vi "Wall avoidance robot.vi"() -> ()   [LabVIEW 2018]
uses:
  <vilib>/myRIO/Common/Instrument Driver Framework/myRIO v1.0/AI/typedefs/AI Channels Enum.ctl
  <vilib>/myRIO/Common/Instrument Driver Framework/myRIO v1.0/AI/typedefs/AI Channels List.ctl
panel:
  in  "Boolean":bool
  out "Sharp IR Distance 2":dbl
  out "Sharp IR Distance":dbl
  out "Speed":T1
  out "Distance":T2
  in  "stop":bool
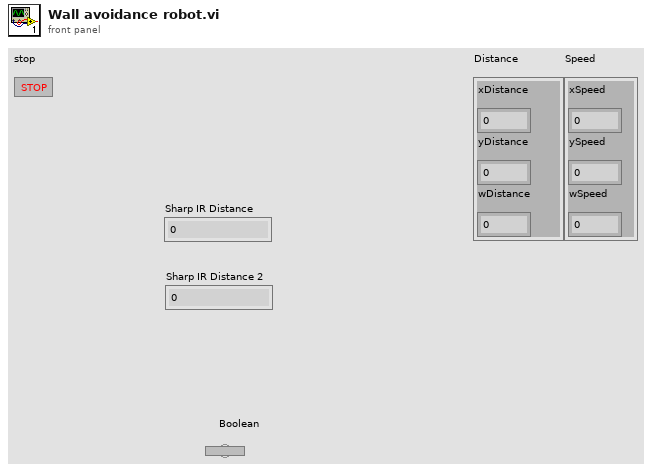
[diagram p1: front panel]
types:
  T1 = cluster{"xSpeed":dbl, "ySpeed":dbl, "wSpeed":dbl}
  T2 = cluster{"xDistance":dbl, "yDistance":dbl, "wDistance":dbl}
  T3 = typedef "AI Channels List.ctl" = T4[]
  T4 = typedef "AI Channels Enum.ctl" = enum16{"Not Connected", "AudioIn/Left", "AudioIn/Right", "C/AI0", "C/AI1", "A/AI0", "A/AI1", "A/AI2", "A/AI3", "A/AI4", "A/AI5", "A/AI6", "A/AI7", "B/AI0", "B/AI1", "B/AI2", "B/AI3", "B/AI4", "B/AI5", "B/AI6", "B/AI7", "AI/AI0", "AI/AI1", "AI/AI2", "AI/AI3", "A/AI0 (DIFF)", "A/AI1 (DIFF)", "A/AI2 (DIFF)", "A/AI3 (DIFF)", "B/AI0 (DIFF)", "B/AI1 (DIFF)", "B/AI2 (DIFF)", "B/AI3 (DIFF)"}
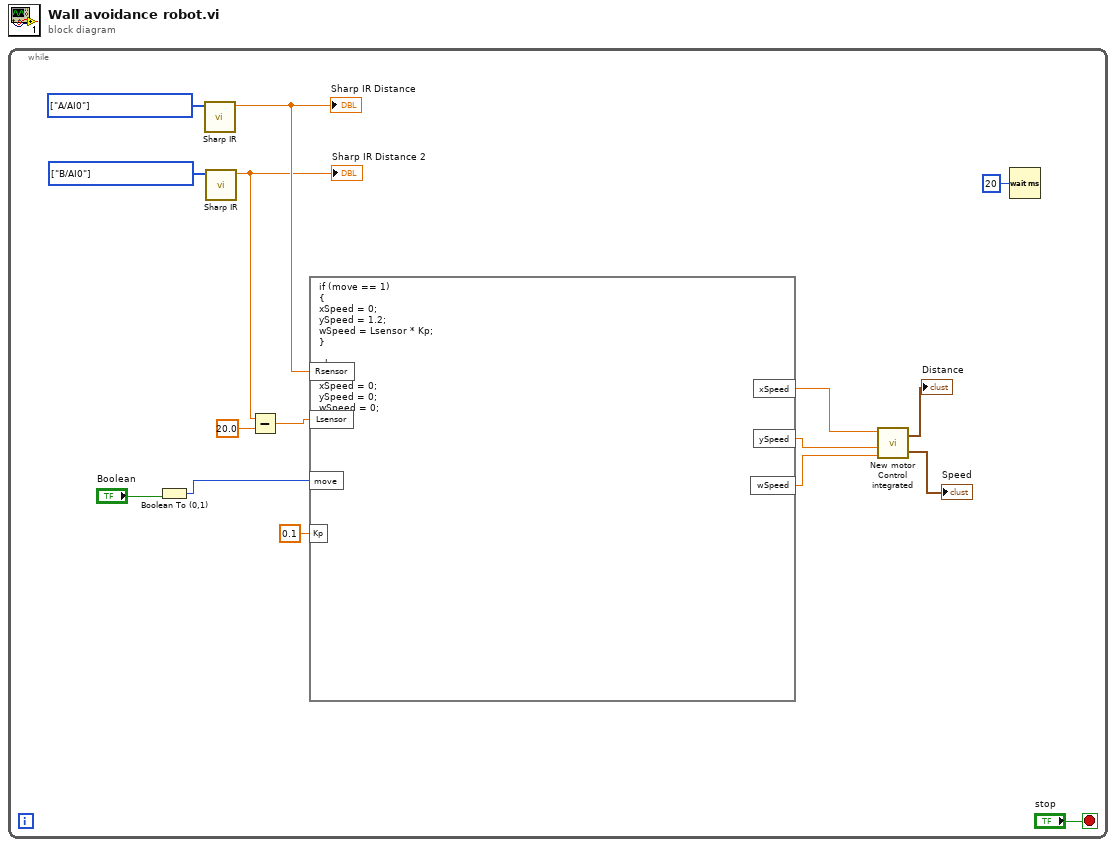
[diagram p0: block diagram]
diagram:
  n1 = while {
    stop <- "stop" stop-if-true
    w8 = T3 [enum."B/AI0"] items=["Not Connected", "AudioIn/Left", "AudioIn/Right", "C/AI0", "C/AI1", "A/AI0", "A/AI1", "A/AI2", "A/AI3", "A/AI4", "A/AI5", "A/AI6", "A/AI7", "B/AI0", "B/AI1", "B/AI2", "B/AI3", "B/AI4", "B/AI5", "B/AI6", "B/AI7", "AI/AI0", "AI/AI1", "AI/AI2", "AI/AI3", "A/AI0 (DIFF)", "A/AI1 (DIFF)", "A/AI2 (DIFF)", "A/AI3 (DIFF)", "B/AI0 (DIFF)", "B/AI1 (DIFF)", "B/AI2 (DIFF)", "B/AI3 (DIFF)"] ("AI Channel")
    w9 = T3 [enum."A/AI0"] items=["Not Connected", "AudioIn/Left", "AudioIn/Right", "C/AI0", "C/AI1", "A/AI0", "A/AI1", "A/AI2", "A/AI3", "A/AI4", "A/AI5", "A/AI6", "A/AI7", "B/AI0", "B/AI1", "B/AI2", "B/AI3", "B/AI4", "B/AI5", "B/AI6", "B/AI7", "AI/AI0", "AI/AI1", "AI/AI2", "AI/AI3", "A/AI0 (DIFF)", "A/AI1 (DIFF)", "A/AI2 (DIFF)", "A/AI3 (DIFF)", "B/AI0 (DIFF)", "B/AI1 (DIFF)", "B/AI2 (DIFF)", "B/AI3 (DIFF)"] ("AI Channel")
    n2 = Boolean To (0,1)(Boolean="Boolean") -> (0, 1=w5:i16)
    n3 = call <vilib>:"Sharp IR.vi"("AI Channel"=w9) -> ("Sharp IR Distance"=w7:dbl)  [unwired: 8 in, 2 out]
    "Sharp IR Distance" <- w7
    n4 = call <vilib>:"Sharp IR.vi"("AI Channel"=w8) -> ("Sharp IR Distance"=w4:dbl)  [unwired: 8 in, 2 out]
    "Sharp IR Distance 2" <- w4
    n5 = Subtract(x=w4, y=20.0) -> (x-y=w2:dbl)
    n6 = formula code="if (move == 1)\n{\nxSpeed = 0;\nySpeed = 1.2;\nwSpeed = Lsensor * Kp;\n}\n\nelse\n{\nxSpeed = 0;\nySpeed = 0;\nwSpeed = 0;\n}"("Rsensor"=w7, "Lsensor"=w2, "move"=w5, "Kp"=0.1 ("input variable")) -> ("xSpeed"=w14:dbl, "ySpeed"=w15:dbl, "wSpeed"=w13:dbl)
    n7 = call "New motor Control integrated.vi"("wTargetSpeed"=w13, "yTargetSpeed"=w15, "Reset Encoders"=w14) -> ("Speed"=→"Speed":T1, "Distance"=→"Distance":T2)  [unwired: 1 in]
    n8 = Wait (ms)(milliseconds to wait=u32 20) -> ()  [unwired: 1 out]
  }
